vi "Application Settings Updated.vi"(8 "error in (no error)":errorcluster, 10 "Reply Payload":T1={"Settings"={"Signal Type"=enum."Sine Wave", "Calibration Array"=[], "Log File Base Path"=path "", "EEG Channels"={"16 EEG Channels"=[], "Gain"=24}, "Soft Trig enum"=enum."Disable Soft Trigger", "Montage selection"={"Montages Ref"=refnum, "Selected Montage Number"=0, "Montages Names"=[]}, "LSL En enum"=enum."LSL Disabled"}, "error"={"status"=FALSE, "code"=0, "source"=""}} {"Settings"."EEG Channels"."16 EEG Channels"."Channel No" step=1}) -> (0 "error out":errorcluster)   [LabVIEW 2019, in "Settings Editor.lvlib"]
doc: "Request Settings Editor to return the latest settings. The Settings Editor can send the applications settings as a reply or via broadcast.\n_____\nCreated using Delacor QMH Event Scripter 4.1.0.75.\n_____\nBased on DQMH Project Template 6.1.0.94."
uses:
  Settings Editor.lvlib
  Update Application Settings (Reply Payload)--cluster.ctl
  Settings--cluster.ctl
  Acquisition/Signal Type--enum.ctl
  Acquisition/Calibration Values--cluster.ctl
  CML Shared/EEG Channel Settings.ctl
  Acquisition/Acquisition.lvlib
  CML Shared/CML Shared.lvlib
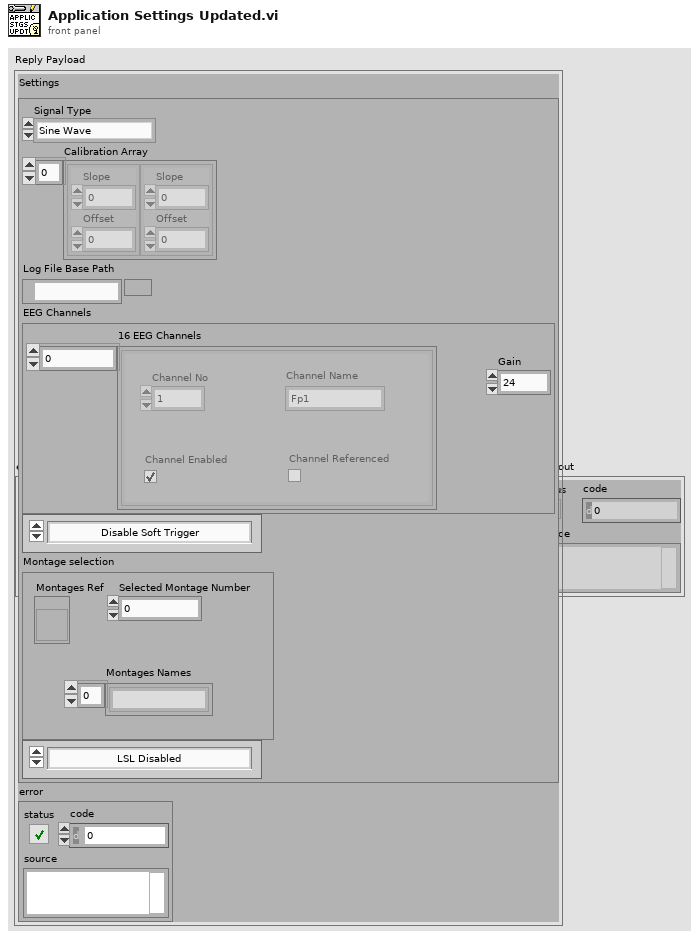
[diagram p1: front panel]
types:
  T1 = typedef "Settings Editor.lvlib/Update Application Settings (Reply Payload)--cluster.ctl" = cluster{"Settings":T2, "error":errorcluster}
  T2 = typedef "Settings Editor.lvlib/Settings--cluster.ctl" = cluster{"Signal Type":T3, "Calibration Array":T4[], "Log File Base Path":path, "EEG Channels":T5, "Soft Trig enum":enum16{"Disable Soft Trigger", "Enable Soft Trigger"}, "Montage selection":cluster{"Montages Ref":refnum<vi>, "Selected Montage Number":u8, "Montages Names":string[]}, "LSL En enum":enum16{"LSL Disabled", "LSL Enabled"}}
  T3 = typedef "Acquisition.lvlib/Signal Type--enum.ctl" = enum16{"Sine Wave", "Square with Noise"}
  T4 = typedef "Acquisition.lvlib/Calibration Values--cluster.ctl" = cluster{"Slope":dbl, "Offset":dbl}
  T5 = typedef "CML Shared.lvlib/EEG Channel Settings.ctl" = cluster{"16 EEG Channels":cluster{"Channel Name":string, "Channel No":u8, "Channel Enabled":bool, "Channel Referenced":bool}[], "Gain":u8}
  T6 = typedef "Settings Editor.lvlib/Broadcast Events--cluster.ctl" = cluster{"Module Did Init":refnum<user-event>, "Status Updated":refnum<user-event>, "Error Reported":refnum<user-event>, "Module Did Stop":refnum<user-event>, "Update Module Execution Status":refnum<user-event>, "Application Settings Updated":refnum<user-event>}
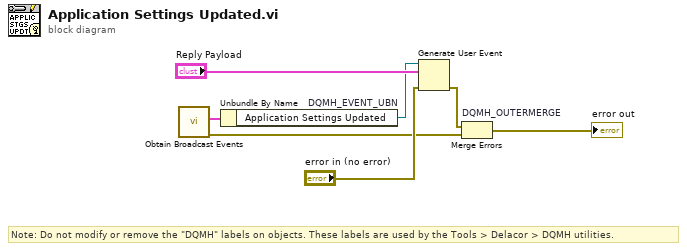
[diagram p0: block diagram]
diagram:
  # "Note: Do not modify or remove the \"DQMH\" labels on objects. These labels are used by the Tools > Delacor > DQMH utilities."
  n1 = call "Obtain Broadcast Events.vi"() -> ("error out"=w2:errorcluster, "Settings Editor Broadcast Events"=w1:T6)  [unwired: 10 in]
  n2 = Unbundle By Name "DQMH_EVENT_UBN"(w1) -> ("Application Settings Updated"=w4:refnum<user-event>)
  n3 = Generate User Event(user event=w4, event data cluster="Reply Payload", error in="error in (no error)") -> (error out=w3:errorcluster)  [unwired: 1 in, 1 out]
  n4 = Merge Errors "DQMH_OUTERMERGE"(w3, w2) -> (→"error out":errorcluster)
